vi "Session Registration Keys.vi"() -> (3 "register annotation keys":string[](array[string]))   [LabVIEW 2021, in "NI Session Management V1 Client.lvlib" / "Session Reservation.lvclass"]
uses:
  Session Reservation.lvclass
  Session Reservation.lvclass/Session Reservation.ctl
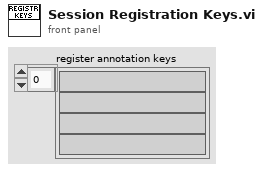
[diagram p1: front panel]
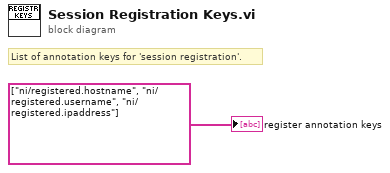
[diagram p0: block diagram]
diagram:
  # "List of annotation keys for 'session registration'."
  "register annotation keys" <- string[] ["ni/registered.hostname", "ni/registered.username", "ni/registered.ipaddress"] ("reserve annotation keys")
